vi "流程写入.vi"(11 "添加的路径":path) -> ()   [LabVIEW 2016]
uses:
  <vilib>/Utility/miscctls.llb/LVPointTypeDef.ctl
panel:
  in  "清洗反应杯":bool
  in  "清洗管路":bool
  in  "填充管路":bool
  in  "加标回收":bool
  in  "平行样":bool
  in  "关闭":bool
  out "字符串":string
  in  "跨度核查":bool
  in  "标样核查":bool
  in  "空白测试":bool
  in  "零点核查":bool
  in  "水样测量":bool=TRUE
  in  "写入":bool
  in  "参数下拉列表":u16(ring)=21 items=["总磷"=0, "总氮"=1, "CODMn"=21]
  in  "量程下拉列表":enum16{"低量程", "高量程"}(ring)
  # "请选择要写入的流程"
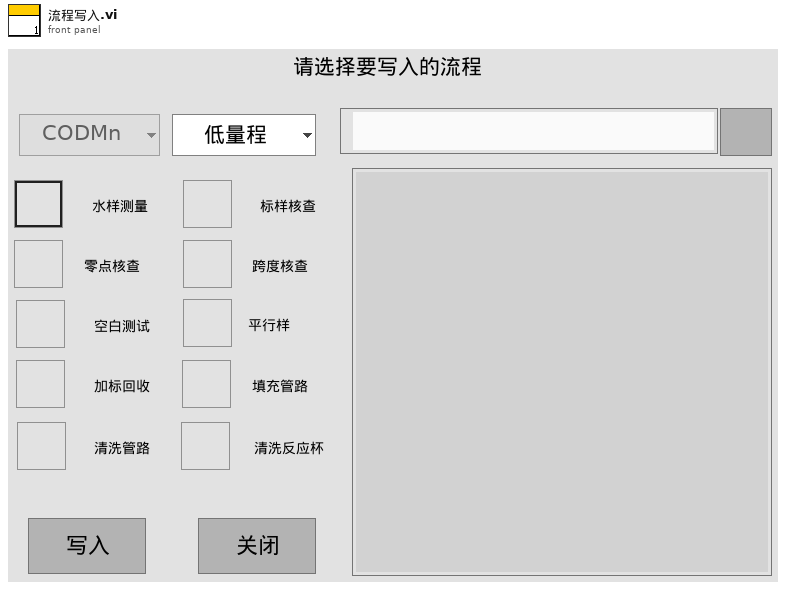
[diagram p1: front panel]
types:
  T1 = typedef "LVPointTypeDef.ctl" = cluster{"Horizontal":i16, "Vertical":i16}
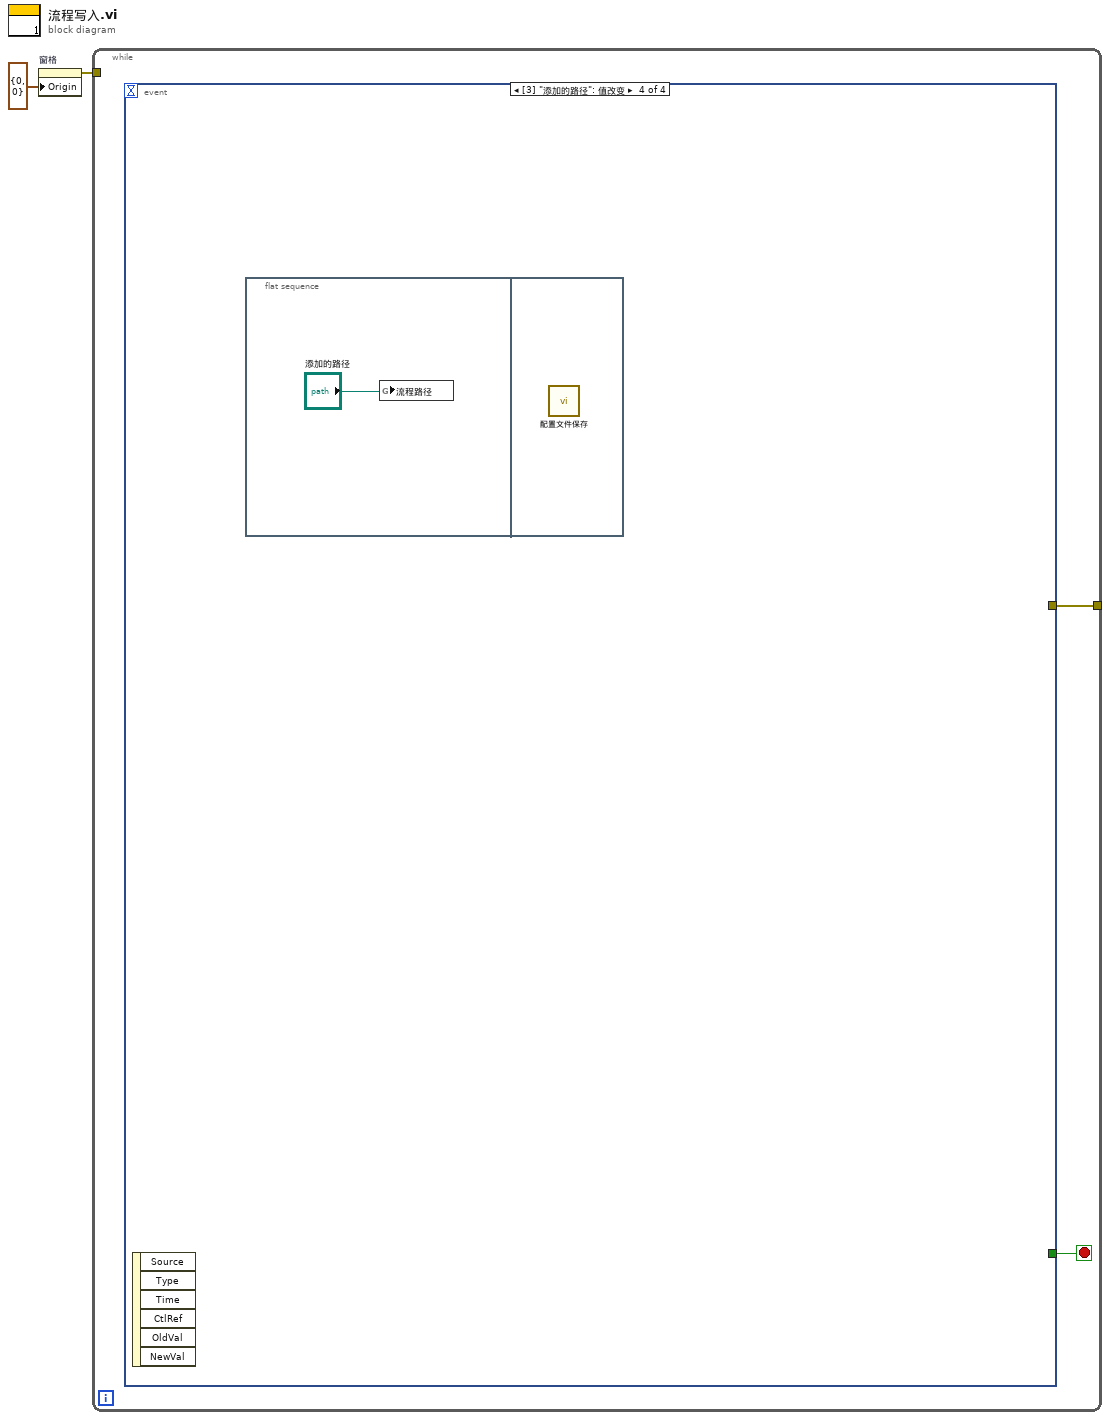
[diagram p0: block diagram]
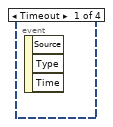
[diagram p2: hidden frame]
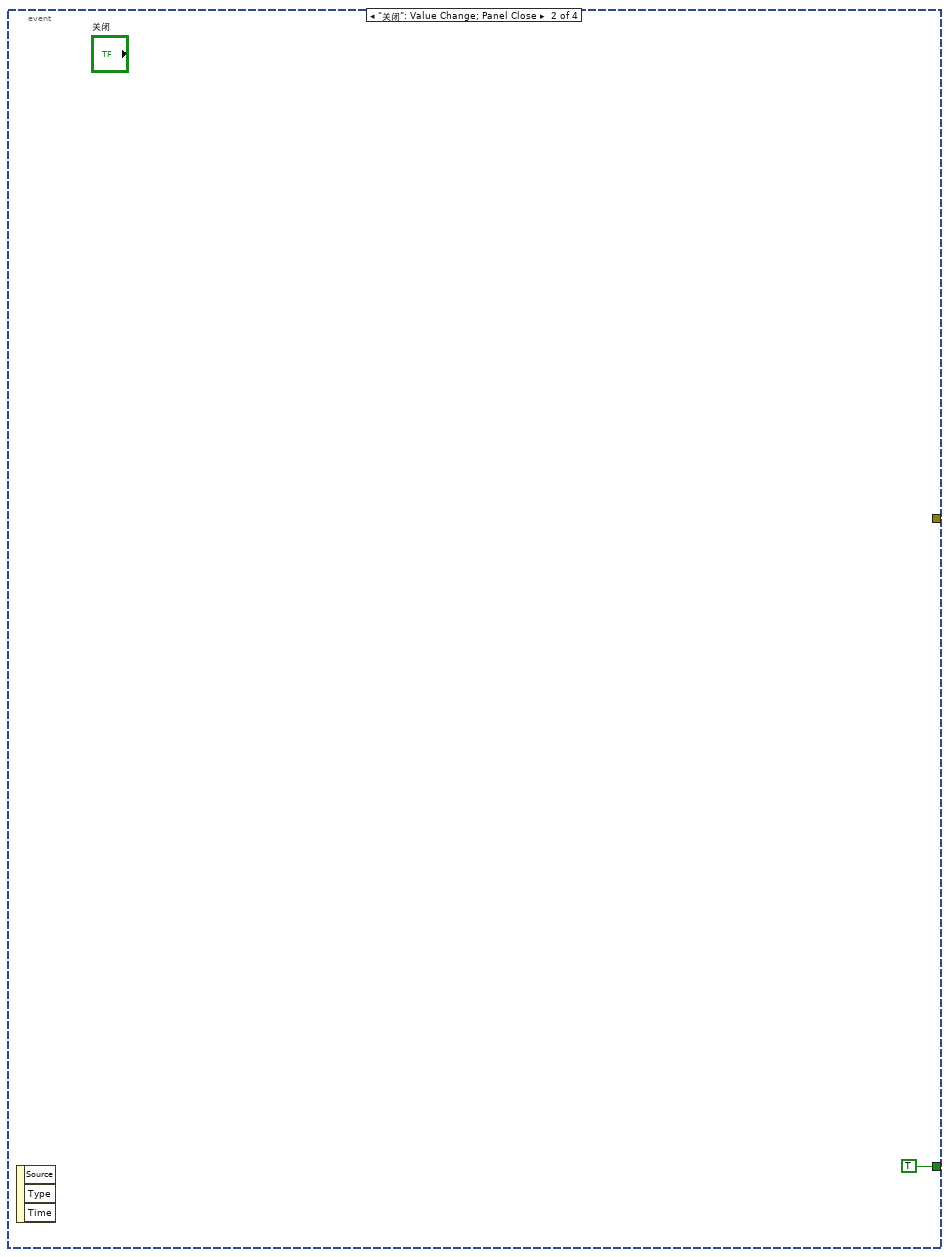
[diagram p3: hidden frame]
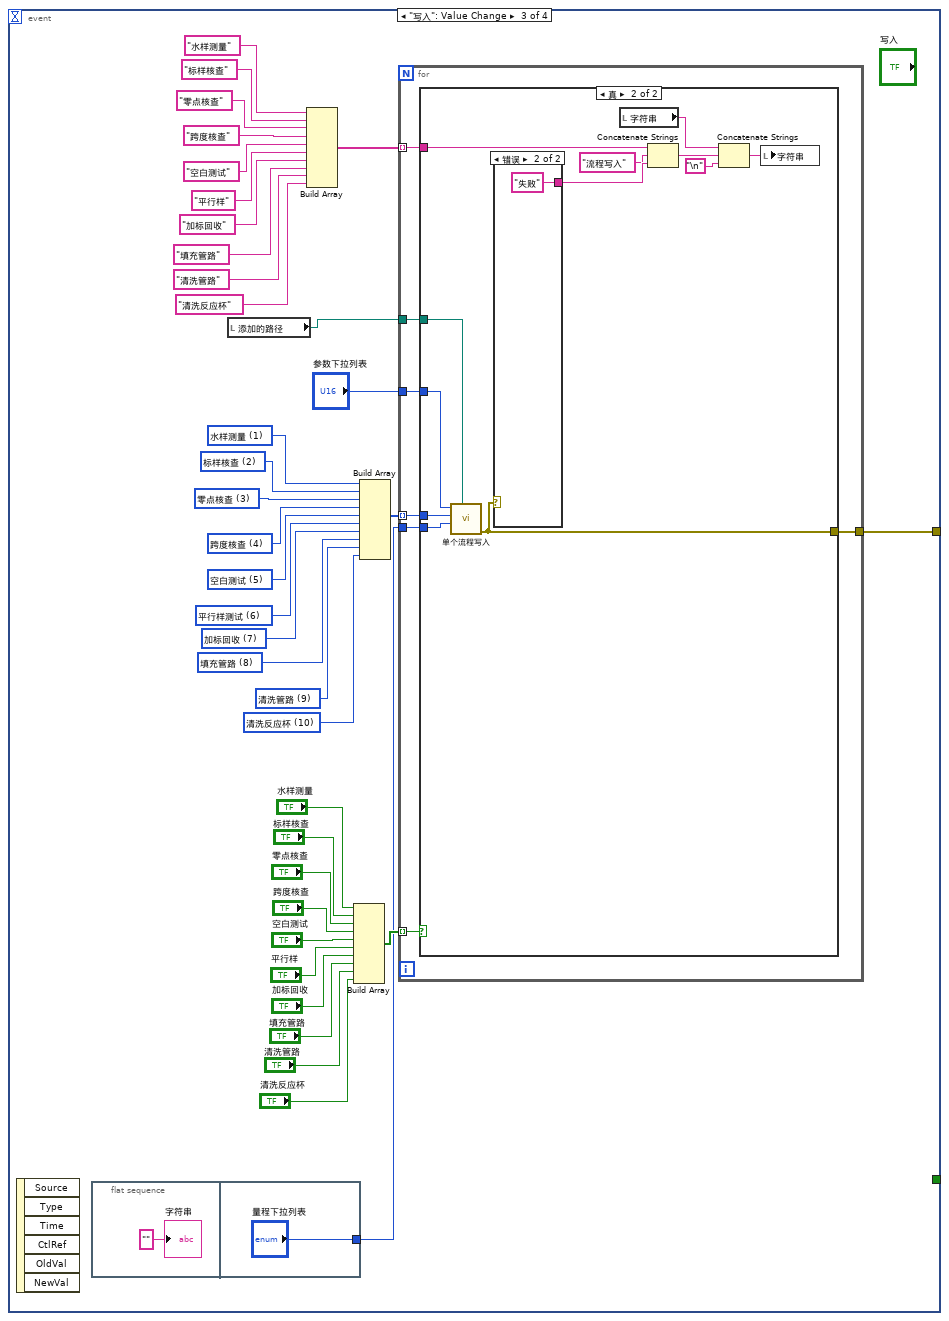
[diagram p4: hidden frame]
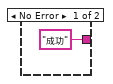
[diagram p6: hidden frame]
diagram:
  n1 = property on="窗格" class="Pane"("Origin"=T1 {"Horizontal"=0, "Vertical"=0} ("原点")) -> (error out=w1:errorcluster)  [unwired: 2 in, 1 out]
  n2 = while {
    tunnel: w1 -> [_]
    tunnel: [w3] -> _
    stop <- w4 stop-if-true
    n3 = event shown="[3] \"添加的路径\": 值改变" {
      selector: _ -> [_ _ _ _]
      dyn-events: _ -> [_ _ _ _]
      timeout: _ -> [_ _ _ _]
      tunnel: [_ TRUE _ _] -> w4
      tunnel: [_ _ w22 _] -> w3
      event Timeout {
        n4 = event-data() -> ()  [unwired: 1 in, 3 out]
      }
      event "关闭": Value Change; Panel Close {
        n5 = event-data() -> ()  [unwired: 1 in, 3 out]
      }
      event "写入": Value Change {
        w18 = u16 10 items=["", "水样测量", "标样核查", "零点核查", "跨度核查", "空白测试", "平行样测试", "加标回收", "填充管路", "清洗管路", "清洗反应杯"] ("测量模式")
        w16 = u16 9 items=["", "水样测量", "标样核查", "零点核查", "跨度核查", "空白测试", "平行样测试", "加标回收", "填充管路", "清洗管路", "清洗反应杯"] ("测量模式")
        w17 = u16 8 items=["", "水样测量", "标样核查", "零点核查", "跨度核查", "空白测试", "平行样测试", "加标回收", "填充管路", "清洗管路", "清洗反应杯"] ("测量模式")
        w35 = u16 7 items=["", "水样测量", "标样核查", "零点核查", "跨度核查", "空白测试", "平行样测试", "加标回收", "校零", "校标"] ("测量模式")
        w34 = u16 6 items=["", "水样测量", "标样核查", "零点核查", "跨度核查", "空白测试", "平行样测试", "加标回收", "校零", "校标"] ("测量模式")
        w33 = u16 5 items=["", "水样测量", "标样核查", "零点核查", "跨度核查", "空白测试", "平行样测试", "加标回收", "校零", "校标"] ("测量模式")
        w32 = u16 4 items=["", "水样测量", "标样核查", "零点核查", "跨度核查", "空白测试", "平行样测试", "加标回收", "校零", "校标"] ("测量模式")
        w10 = u16 2 items=["", "水样测量", "标样核查", "零点核查", "跨度核查", "空白测试", "平行样测试", "加标回收", "校零", "校标"] ("测量模式")
        w9 = u16 3 items=["", "水样测量", "标样核查", "零点核查", "跨度核查", "空白测试", "平行样测试", "加标回收", "校零", "校标"] ("测量模式")
        w31 = u16 1 items=["", "水样测量", "标样核查", "零点核查", "跨度核查", "空白测试", "平行样测试", "加标回收", "校零", "校标"] ("测量模式")
        n6 = event-data() -> ()  [unwired: 1 in, 6 out]
        n7 = flat-sequence {
          tunnel: ["量程下拉列表"] -> w23
          frame #0 {
            "字符串" <- ""
          }
          frame #1 {
          }
        }
        n8 = local read "添加的路径"() -> (w6:path)
        n9 = Build Array("水样测量", "标样核查", "零点核查", "跨度核查", "空白测试", "平行样", "加标回收", "填充管路", "清洗管路", "清洗反应杯") -> (w42:string[])
        n10 = Build Array("水样测量", "标样核查", "零点核查", "跨度核查", "空白测试", "平行样", "加标回收", "填充管路", "清洗管路", "清洗反应杯") -> (w30:bool[])
        n11 = Build Array(w31, w10, w9, w32, w33, w34, w35, w17, w16, w18) -> (w41:u16[])
        n12 = for {
          tunnel: w30 -> [w49] mode=indexing
          tunnel: w41 -> [w47] mode=indexing
          tunnel: w42 -> [w48] mode=indexing
          tunnel: w6 -> [w46]
          tunnel: "参数下拉列表" -> [w45]
          tunnel: w23 -> [w44]
          tunnel: [w43] -> w22
          n13 = case shown="真" w49 {
            tunnel: w48 -> [_ w55]
            tunnel: w47 -> [_ w50]
            tunnel: w46 -> [_ w54]
            tunnel: w45 -> [_ w53]
            tunnel: w44 -> [_ w52]
            tunnel: [_ w51] -> w43
            frame False {
            }
            frame True {
              n14 = call "单个流程写入.vi"("添加的路径"=w54, "量程"=w52, "测量模式"=w50, "测量参数"=w53) -> ("error out"=w51:errorcluster)  [unwired: 6 in, 1 out]
              n15 = case shown="错误" w51 {
                tunnel: ["成功" "失败"] -> w58
                frame No Error {
                }
                frame Error {
                }
              }
              n16 = local read "字符串"() -> (w56:string)
              n17 = Concatenate Strings(w55, "流程写入", w58) -> (w59:string)
              n18 = Concatenate Strings(w56, w59, "\n") -> (w61:string)
              n19 = local write "字符串"(w61) -> ()
            }
          }
        }
      }
      event "添加的路径": Value Change {
        n20 = event-data() -> ()  [unwired: 1 in, 6 out]
        n21 = flat-sequence {
          frame #0 {
            n22 = global write "挥发酚断电保存全局变量.vi" "流程路径"("添加的路径") -> ()
          }
          frame #1 {
            n23 = call "配置文件保存.vi"() -> ()  [unwired: 12 in]
          }
        }
      }
    }
  }
